vi "color map in histogram.vi"() -> ()   [LabVIEW 2015]
uses:
  Type Defs/Color Map.ctl
panel:
  in  "Boolean":bool
  out "Histogram":T1(graph)
  in  "Color Map":T2=enum."Green"
  out "Intensity Graph":dbl[][](graph)
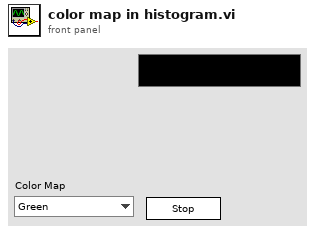
[diagram p1: front panel]
types:
  T1 = cluster{"X Values":dbl[], "Histogram: h(x)":i32[]}
  T2 = typedef "Color Map.ctl" = enum16{"Boring", "Fire", "Crazy", "Asylum", "Cubehelix", "Red", "Green", "Blue"}
  T3 = typedef "LVRectTypeDef.ctl" = cluster{"Left":i16, "Top":i16, "Right":i16, "Bottom":i16}
  T4 = cluster{"Cursor.Cursor X":dbl, "Cursor.Cursor Position:Cursor X":dbl}
  T5 = typedef "LVPoint32TypeDef.ctl" = cluster{"Horizontal":i32, "Vertical":i32}
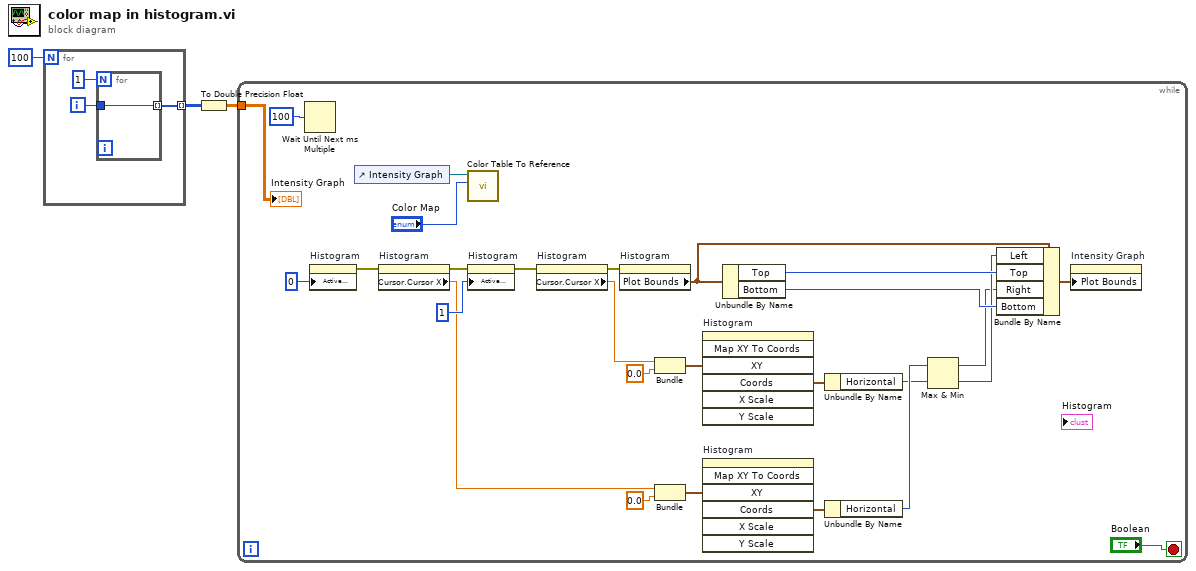
[diagram p0: block diagram]
diagram:
  n1 = for {
    N: 100 -> [_]
    tunnel: [w5] -> w2 mode=indexing
    i -> [w6]
    n2 = for {
      N: 1 -> [_]
      tunnel: w6 -> [w7]
      tunnel: [w7] -> w5 mode=indexing
    }
  }
  n3 = To Double Precision Float(number=w2) -> (double precision float=w1:dbl[][])
  n4 = while {
    tunnel: w1 -> [w8]
    stop <- "Boolean" stop-if-true
    n5 = Wait Until Next ms Multiple(millisecond multiple=u32 100) -> ()  [unwired: 1 out]
    n6 = property on="Histogram" class="XYGraph (strict)"("Active Cursor"=u32 0) -> (error out=w29:errorcluster)  [unwired: 2 in, 1 out]
    n7 = control-ref of="Intensity Graph"() -> (w33:refnum<vi>)
    n8 = property on="Histogram" class="XYGraph (strict)"(error in=w29) -> (error out=w26:errorcluster, "Cursor.Cursor X"=w21:dbl)  [unwired: 1 in, 1 out]
    n9 = call "Color Table To Reference.vi"("Color Map"="Color Map", "Intensity Graph Reference"=w33) -> ()  [unwired: 10 in]
    n10 = property on="Histogram" class="XYGraph (strict)"(error in=w26, "Active Cursor"=u32 1) -> (error out=w28:errorcluster)  [unwired: 1 in, 1 out]
    n11 = property on="Histogram" class="XYGraph (strict)"(error in=w28) -> (error out=w25:errorcluster, "Cursor.Cursor X"=w15:dbl)  [unwired: 1 in, 1 out]
    n12 = property on="Histogram" class="XYGraph (strict)"(error in=w25) -> ("Plot Bounds"=w24:T3)  [unwired: 1 in, 2 out]
    n13 = Bundle("Cursor.Cursor X"=w15, "Cursor.Cursor Position:Cursor X"=0.0) -> (w14:T4)  [unwired: 1 in]
    n14 = Bundle("Cursor.Cursor X"=w21, "Cursor.Cursor Position:Cursor X"=0.0) -> (w19:T4)  [unwired: 1 in]
    n15 = invoke on="Histogram" class="XYGraph (strict)" method="Map XY To Coords"("XY"=w14) -> ("Coords"=w13:T5)  [unwired: 6 in, 6 out]
    n16 = invoke on="Histogram" class="XYGraph (strict)" method="Map XY To Coords"("XY"=w19) -> ("Coords"=w18:T5)  [unwired: 6 in, 6 out]
    n17 = Unbundle By Name(w24) -> ("Top"=w23:i16, "Bottom"=w22:i16)
    n18 = Unbundle By Name(w13) -> ("Horizontal"=w12:i32)
    n19 = Unbundle By Name(w18) -> ("Horizontal"=w17:i32)
    n20 = Max & Min(x=w17, y=w12) -> (max(x,y)=w10:i32, min(x,y)=w11:i32)
    n21 = Bundle By Name(cluster=w24, "Left"=w11, "Top"=w23, "Right"=w10, "Bottom"=w22) -> (w9:T3)
    n22 = property on="Intensity Graph" class="IntGraph (strict)"("Plot Bounds"=w9) -> ()  [unwired: 2 in, 2 out]
    "Intensity Graph" <- w8
  }
